vi "Event-Driven State Machine Property Nodes.vi"() -> ()   [LabVIEW 2020]
uses:
  support/States.ctl
  support/State Machine Data.ctl
  <vilib>/DAQmx/read.llb/DAQmx Read (Analog 2D DBL NChan NSamp).vi
  <vilib>/DAQmx/write.llb/DAQmx Write (Analog DBL 1Chan 1Samp).vi
  <vilib>/DAQmx/create/channels.llb/DAQmx Create Channel (AI-Voltage-Basic).vi
  <vilib>/DAQmx/configure/timing.llb/DAQmx Timing (Sample Clock).vi
  <vilib>/DAQmx/miscellaneous.llb/DAQmx Fill In Error Info.vi
  <vilib>/Utility/file.llb/Write Delimited Spreadsheet (DBL).vi
  <vilib>/DAQmx/create/channels.llb/DAQmx Create Channel (AO-Voltage-Basic).vi
panel:
  in  "AO Voltage Channel":tag="PCI-6221/ao1"
  in  "Generate Stimulus":bool
  out "RMS Results Per Channel":dbl[](array[numeric])
  out "Threshold exceeded?":bool
  in  "Acquire":bool
  in  "Samples per channel":i32=100
  in  "Sample Rate (Hz)":dbl=1000.0
  in  "AI Voltage Channel":tag="PCI-6221/ai0, PCI-6221/ai2:3"
  in  "Threshold (rms)":dbl=1.0
  in  "Clear":bool
  in  "Exit":bool
  out "Graph":dbl[][](graph)
  # "Analysis"
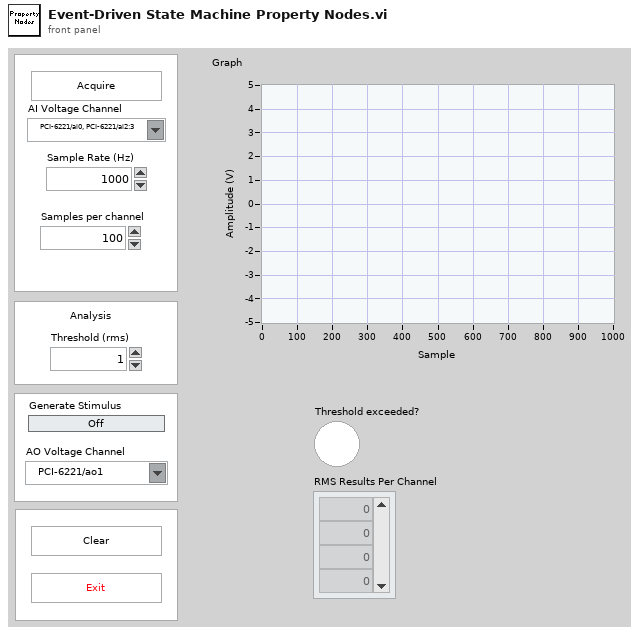
[diagram p1: front panel]
types:
  T1 = typedef "State Machine Data.ctl" = cluster{"Acquisition Data":dbl[][], "Stimulus Value":bool}
  T2 = typedef "States.ctl" = enum16{"Initialize", "Wait for Event", "Acquire", "Analyze", "Log", "Clear", "Update UI", "Update Stumulus", "Exit"}
  T3 = enum8{"Enabled", "Disabled", "Disabled and Grayed Out"}
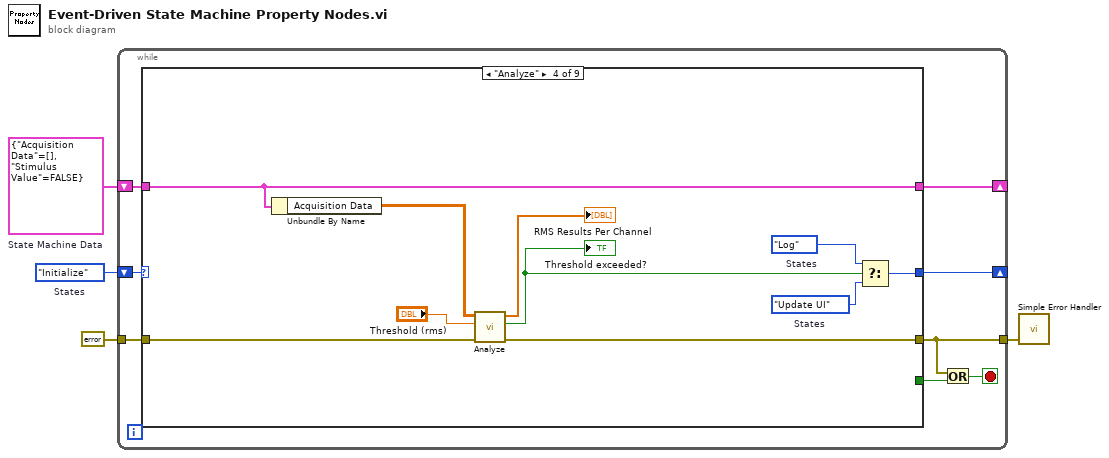
[diagram p0: block diagram]
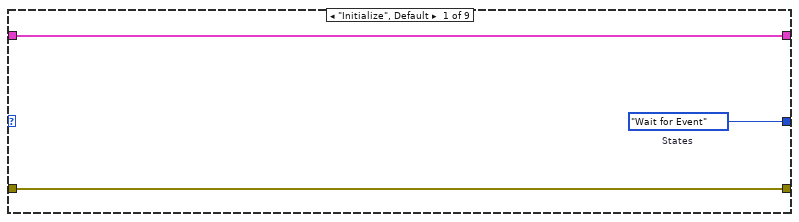
[diagram p2: hidden frame]
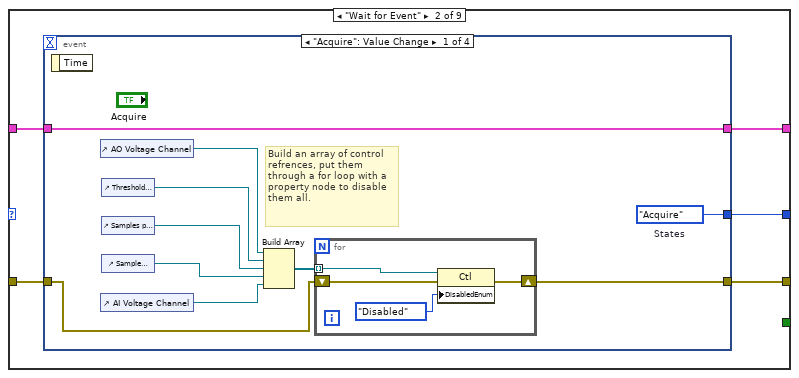
[diagram p3: hidden frame]
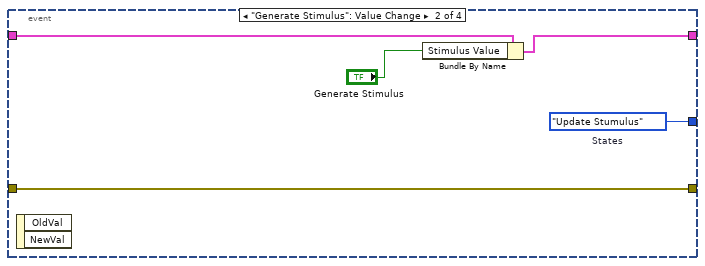
[diagram p4: hidden frame]
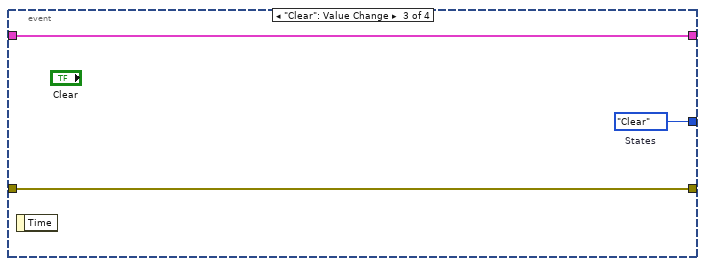
[diagram p5: hidden frame]
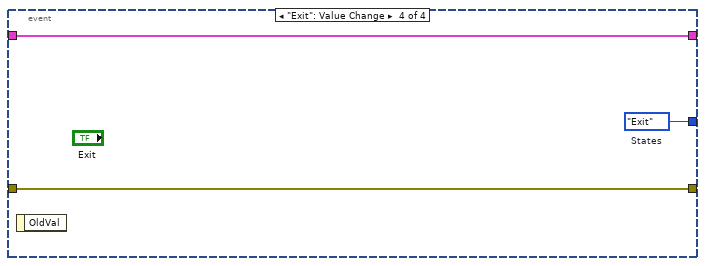
[diagram p6: hidden frame]
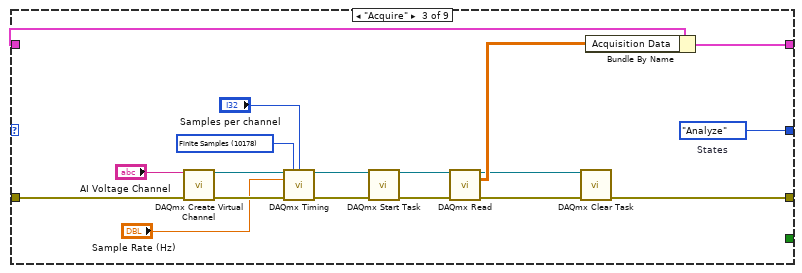
[diagram p7: hidden frame]
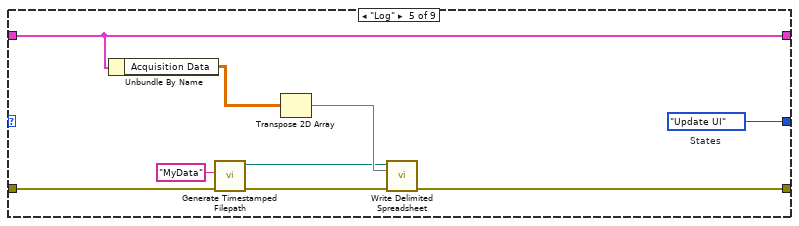
[diagram p8: hidden frame]
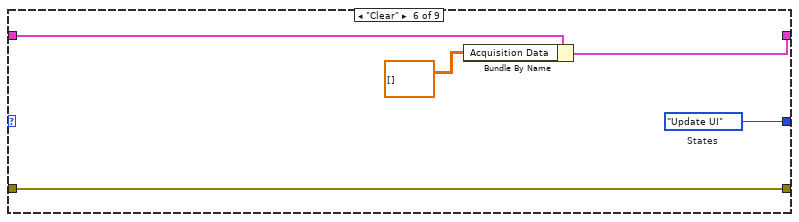
[diagram p9: hidden frame]
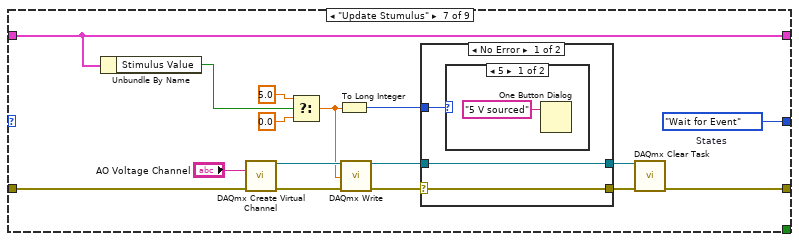
[diagram p10: hidden frame]
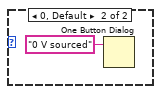
[diagram p11: hidden frame]
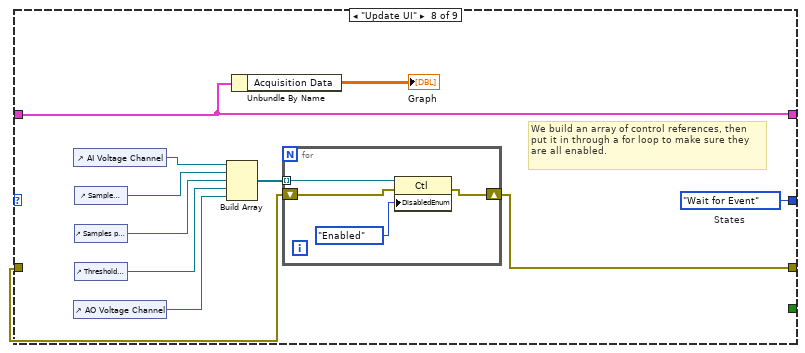
[diagram p13: hidden frame]
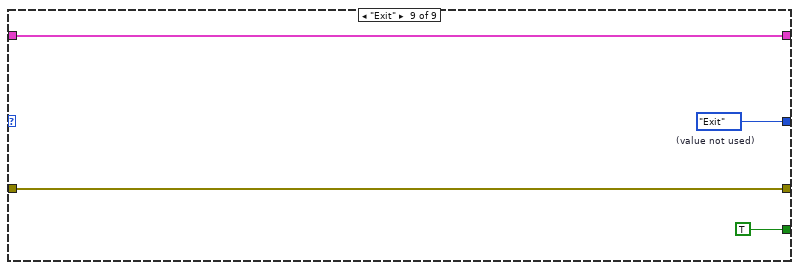
[diagram p14: hidden frame]
diagram:
  w4 = T1 {"Acquisition Data"=[], "Stimulus Value"=FALSE}  # State Machine Data
  w3 = States."Initialize"  # States
  n1 = while {
    tunnel: errorcluster {"status"=FALSE, "code"=0, "source"=""} ("error constant") -> [w11]
    tunnel: [w7] -> w1
    shift-right: [w9] -> _
    shift-left: w4 -> [w10]
    shift-right: [w8] -> _
    shift-left: w3 -> [w12]
    stop <- w6 stop-if-true
    n2 = case shown="\"Analyze\"" w12 {
      tunnel: w11 -> [w15 w18 w63 w72 w81 w87 w93 w111 w128]
      tunnel: [w15 w17 w58 w71 w75 w87 w92 w112 w128] -> w7
      tunnel: [w14 w19 w55 w73 w82 w85 w103 w119 w129] -> w9
      tunnel: w10 -> [w14 w20 w56 w73 w82 w86 w103 w119 w129]
      tunnel: [w13 w16 w57 w67 w74 w83 w94 w121 w126] -> w8
      tunnel: [_ _ _ _ _ _ _ _ TRUE] -> w5
      frame "Initialize", Default {
        w13 = States."Wait for Event"  # States
      }
      frame "Wait for Event" {
        n3 = event shown="[0] \"Acquire\": Value Change" {
          selector: _ -> [_ _ _ _]
          dyn-events: _ -> [_ _ _ _]
          timeout: _ -> [_ _ _ _]
          tunnel: w20 -> [w29 w39 w42 w44]
          tunnel: [w29 w38 w42 w44] -> w19
          tunnel: w18 -> [w21 w35 w41 w45]
          tunnel: [w22 w35 w41 w45] -> w17
          tunnel: [w30 w36 w40 w43] -> w16
          event "Acquire": Value Change {
            w30 = States."Acquire"  # States
            # "Build an array of control refrences, put them through a for loop with a property node to disable them all."
            n4 = event-data() -> ()  [unwired: 1 in, 1 out]
            n5 = control-ref of="AO Voltage Channel"() -> (w28:refnum<vi>)
            n6 = control-ref of="AI Voltage Channel"() -> (w24:refnum<vi>)
            n7 = control-ref of="Threshold (rms)"() -> (w27:refnum<vi>)
            n8 = control-ref of="Samples per channel"() -> (w26:refnum<vi>)
            n9 = control-ref of="Sample Rate (Hz)"() -> (w25:refnum<vi>)
            n10 = Build Array(w28, w27, w26, w25, w24) -> (w23:refnum<vi>[])
            n11 = for {
              tunnel: w23 -> [w34] mode=indexing
              shift-right: [w31] -> w22
              shift-left: w21 -> [w33]
              n12 = property class="Ctl"(reference=w34, error in=w33, "DisabledEnum"=T3."Disabled" ("Disabled")) -> (error out=w31:errorcluster)  [unwired: 1 out]
            }
          }
          event "Generate Stimulus": Value Change {
            w36 = States."Update Stumulus"  # States
            n13 = event-data() -> ()  [unwired: 1 in, 2 out]
            n14 = Bundle By Name(cluster=w39, "Stimulus Value"="Generate Stimulus") -> (w38:T1)
          }
          event "Clear": Value Change {
            w40 = States."Clear"  # States
            n15 = event-data() -> ()  [unwired: 1 in, 1 out]
          }
          event "Exit": Value Change {
            w43 = States."Exit"  # States
            n16 = event-data() -> ()  [unwired: 1 in, 1 out]
          }
        }
      }
      frame "Acquire" {
        w54 = 10178 items=["Finite Samples"=10178, "Continuous Samples"=10123, "Hardware Timed Single Point"=12522] ("sample mode")
        w57 = States."Analyze"  # States
        n17 = call-poly <vilib>:"DAQmx Create Virtual Channel.vi"("physical channels"="AI Voltage Channel", "error in"=w63) -> ("task out"=w49:refnum<k21>, "error out"=w62:errorcluster)  [unwired: 12 in]
        n18 = call-poly <vilib>:"DAQmx Timing.vi"("task/channels in"=w49, "sample mode"=w54, "samples per channel"="Samples per channel", "rate"="Sample Rate (Hz)", "error in"=w62) -> ("task out"=w48:refnum<k21>, "error out"=w61:errorcluster)  [unwired: 9 in]
        n19 = call <vilib>:"DAQmx Start Task.vi"("task/channels in"=w48, "error in"=w61) -> ("task out"=w47:refnum<k21>, "error out"=w60:errorcluster)  [unwired: 12 in]
        n20 = call-poly <vilib>:"DAQmx Read.vi"("task/channels in"=w47, "error in"=w60) -> ("task out"=w46:refnum<k21>, "data"=w50:dbl[][], "error out"=w59:errorcluster)  [unwired: 11 in]
        n21 = call <vilib>:"DAQmx Clear Task.vi"("task in"=w46, "error in"=w59) -> ("error out"=w58:errorcluster)  [unwired: 13 in]
        n22 = Bundle By Name(cluster=w56, "Acquisition Data"=w50) -> (w55:T1)
      }
      frame "Analyze" {
        w68 = States."Update UI"  # States
        w69 = States."Log"  # States
        n23 = Unbundle By Name(w73) -> ("Acquisition Data"=w70:dbl[][])
        n24 = call "Analyze.vi"("Error In"=w72, "Treshold (rms)"="Threshold (rms)", "N-Channel Data (2D DBL)"=w70) -> ("Error Out"=w71:errorcluster, "Threshold exceeded?"=w64:bool, "N-Channel Data RMS Results"=→"RMS Results Per Channel":dbl[])  [unwired: 5 in, 1 out]
        "Threshold exceeded?" <- w64
        n25 = Select(t=w69, s=w64, f=w68) -> (s? t:f=w67:T2)
      }
      frame "Log" {
        w74 = States."Update UI"  # States
        n26 = Unbundle By Name(w82) -> ("Acquisition Data"=w79:dbl[][])
        n27 = call "Generate Timestamped Filepath.vi"("Error In"=w81, "appended filename"="MyData") -> ("Error Out"=w76:errorcluster, "timestamped relative filepath"=w77:path)  [unwired: 8 in]
        n28 = Transpose 2D Array(2D array=w79) -> (transposed array=w78:dbl[][])
        n29 = call-poly <vilib>:"Write Delimited Spreadsheet.vi"("file path (dialog if empty)"=w77, "2D data"=w78, "error in (no error)"=w76) -> ("error out"=w75:errorcluster)  [unwired: 11 in, 1 out]
      }
      frame "Clear" {
        w83 = States."Update UI"  # States
        n30 = Bundle By Name(cluster=w86, "Acquisition Data"=dbl[][] []) -> (w85:T1)
      }
      frame "Update Stumulus" {
        w94 = States."Wait for Event"  # States
        n31 = Unbundle By Name(w103) -> ("Stimulus Value"=w95:bool)
        n32 = call-poly <vilib>:"DAQmx Create Virtual Channel.vi"("physical channels"="AO Voltage Channel", "error in"=w93) -> ("task out"=w100:refnum<k21>, "error out"=w99:errorcluster)  [unwired: 12 in]
        n33 = Select(t=5.0, s=w95, f=0.0) -> (s? t:f=w97:dbl)
        n34 = To Long Integer(number=w97) -> (32bit integer=w96:i32)
        n35 = call-poly <vilib>:"DAQmx Write.vi"("task/channels in"=w100, "data"=w97, "error in"=w99) -> ("task out"=w90:refnum<k21>, "error out"=w91:errorcluster)  [unwired: 10 in, 1 out]
        n36 = case shown="No Error" w91 {
          selector: w91 -> [w104 w109]
          tunnel: w96 -> [w106 _]
          tunnel: w90 -> [w105 w110]
          tunnel: [w105 w110] -> w89
          tunnel: [w104 w109] -> w88
          frame No Error {
            n37 = case shown="5" w106 {
              frame 5 {
                n38 = One Button Dialog(message="5 V sourced") -> ()  [unwired: 1 in, 1 out]
              }
              frame 0, Default {
                n39 = One Button Dialog(message="0 V sourced") -> ()  [unwired: 1 in, 1 out]
              }
            }
          }
          frame Error {
          }
        }
        n40 = call <vilib>:"DAQmx Clear Task.vi"("task in"=w89, "error in"=w88) -> ("error out"=w92:errorcluster)  [unwired: 13 in]
      }
      frame "Update UI" {
        w121 = States."Wait for Event"  # States
        # "We build an array of control references, then put it in through a for loop to make sure they are all enabled."
        n41 = control-ref of="AI Voltage Channel"() -> (w118:refnum<vi>)
        n42 = control-ref of="AO Voltage Channel"() -> (w114:refnum<vi>)
        n43 = control-ref of="Sample Rate (Hz)"() -> (w117:refnum<vi>)
        n44 = control-ref of="Samples per channel"() -> (w116:refnum<vi>)
        n45 = control-ref of="Threshold (rms)"() -> (w115:refnum<vi>)
        n46 = Build Array(w118, w117, w116, w115, w114) -> (w113:refnum<vi>[])
        n47 = Unbundle By Name(w119) -> ("Acquisition Data"=→"Graph":dbl[][])
        n48 = for {
          tunnel: w113 -> [w125] mode=indexing
          shift-right: [w122] -> w112
          shift-left: w111 -> [w123]
          n49 = property class="Ctl"(reference=w125, error in=w123, "DisabledEnum"=T3."Enabled" ("Disabled")) -> (error out=w122:errorcluster)  [unwired: 1 out]
        }
      }
      frame "Exit" {
        w126 = States."Exit"  # (value not used)
      }
    }
    n50 = Or(x=w7, y=w5) -> (x .or. y?=w6:bool)
  }
  n51 = call <vilib>:"Simple Error Handler.vi"("error in (no error)"=w1) -> ()  [unwired: 4 in, 5 out]
